vi "Prober_MoveToXYZTheta.vi"(6 "Theta location [mdeg]":string="none", 7 "ProbeStationControl in":refnum<class "ProbeStationControl.lvclass">, 8 "error in (no error)":errorcluster, 9 "Z location [µm]":string="none", 10 "Y location [µm]":string="none", 11 "X location [µm]":string="none") -> (0 "error out":errorcluster, 2 "String":string, 3 "ProbeStationControl out":refnum<class "ProbeStationControl.lvclass">)   [LabVIEW 2018, in "ProbeStationControl.lvclass"]
uses:
  ProbeStationControl.lvclass
  ProbeStationControl.lvclass/ProbeStationControl.ctl
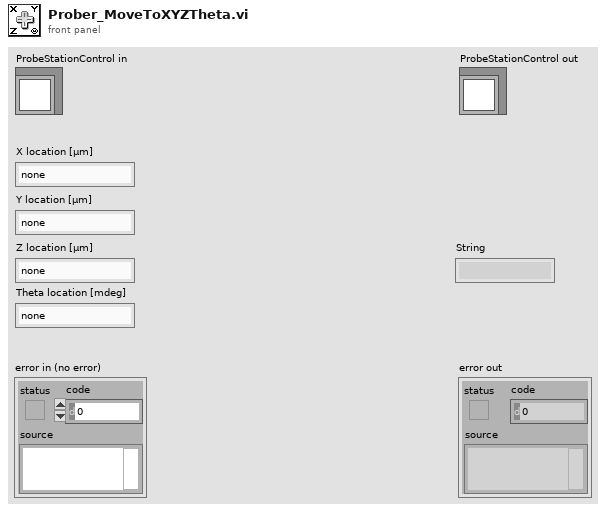
[diagram p1: front panel]
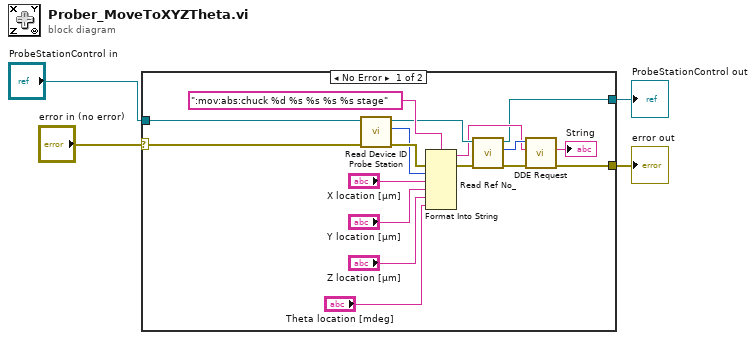
[diagram p0: block diagram]
diagram:
  n1 = case shown="No Error" "error in (no error)" {
    selector: "error in (no error)" -> [w14 w23]
    tunnel: [w19 w23] -> w3
    tunnel: "ProbeStationControl in" -> [w15 w22]
    tunnel: [w5 w22] -> w1
    frame No Error {
      n2 = call "Read Device ID Probe Station.vi"("error in (no error)"=w14, "ProbeStationControl in"=w15) -> ("error out"=w13:errorcluster, "Device ID Probe Station"=w11:u32, "ProbeStationControl out"=w12:refnum<class "ProbeStationControl.lvclass">)  [unwired: 7 in]
      n3 = Format Into String(format string=":mov:abs:chuck %d %s %s %s %s stage", error in=w13, w11, "X location [µm]", "Y location [µm]", "Z location [µm]", "Theta location [mdeg]") -> (resulting string=w6:string, error out=w17:errorcluster)  [unwired: 1 in]
      n4 = call "Read Ref No_.vi"("error in (no error)"=w17, "ProbeStationControl in"=w12) -> ("error out"=w20:errorcluster, "Ref No."=w21:i32, "ProbeStationControl out"=w5:refnum<class "ProbeStationControl.lvclass">)  [unwired: 7 in]
      n5 = call <vilib>:"DDE Request.vi"("error in (no error)"=w20, "item"=w6, "conversation refnum in"=w21) -> ("error out"=w19:errorcluster, "data"=→"String":string)  [unwired: 4 in, 1 out]
    }
    frame Error {
    }
  }
  "error out" <- w3
  "ProbeStationControl out" <- w1
